vi "planta.vi"(8 "yk-2":dbl, 9 "yk-1":dbl, 10 "mk-2":dbl, 11 "mk-1":dbl) -> (2 "yk":dbl)   [LabVIEW 2019]
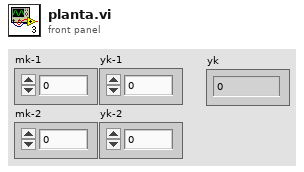
[diagram p1: front panel]
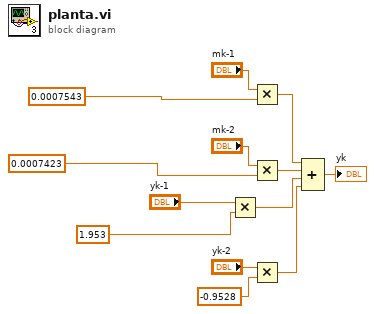
[diagram p0: block diagram]
diagram:
  n1 = Multiply(x="yk-1", y=1.953) -> (x*y=w11:dbl)
  n2 = Multiply(x="mk-1", y=0.0007543) -> (x*y=w13:dbl)
  n3 = Multiply(x="mk-2", y=0.0007423) -> (x*y=w12:dbl)
  n4 = Multiply(x="yk-2", y=-0.9528) -> (x*y=w10:dbl)
  n5 = Compound Arithmetic op=ADD(w13, w12, w11, w10) -> (→"yk":dbl)
